vi "Get Request Type.vi"(8 "error in (no error)":errorcluster, 11 "GetCurrentProgramScene in":refnum<class "GetCurrentProgramScene.lvclass">) -> (0 "error out":errorcluster, 2 "Request Type":string, 3 "GetCurrentProgramScene out":refnum<class "GetCurrentProgramScene.lvclass">)   [LabVIEW 2022 SP3, in "obs-websocket-lv.lvlib" / "GetCurrentProgramScene.lvclass"]
uses:
  GetCurrentProgramScene.lvclass
  GetCurrentProgramScene.lvclass/GetCurrentProgramScene.ctl
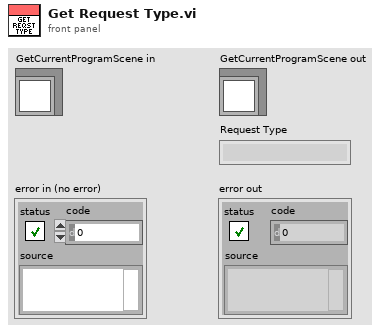
[diagram p1: front panel]
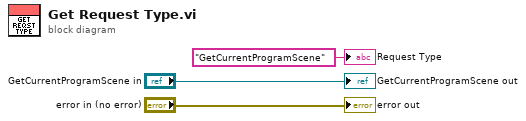
[diagram p0: block diagram]
diagram:
  "error out" <- "error in (no error)"
  "GetCurrentProgramScene out" <- "GetCurrentProgramScene in"
  "Request Type" <- "GetCurrentProgramScene" ("Request Type")
